vi "get_trigger.vi"(8 "error in (no error)":errorcluster, 11 "DAQmxWriteSignals in":refnum<class "SignalWriterMM140725DAQmx.lvclass">) -> (0 "error out":errorcluster, 1 "edge":T1, 2 "digital trigger line":tag, 3 "DAQmxWriteSignals out":refnum<class "SignalWriterMM140725DAQmx.lvclass">, 4 "trigger set?":bool)   [LabVIEW 2010, in "SignalWriterMM140725DAQmx.lvclass"]
uses:
  SignalWriterMM140725DAQmx.lvclass
  trigger_edge_enum.ctl
  SignalWriterMM140725DAQmx.lvclass/SignalWriterMM140725DAQmx.ctl
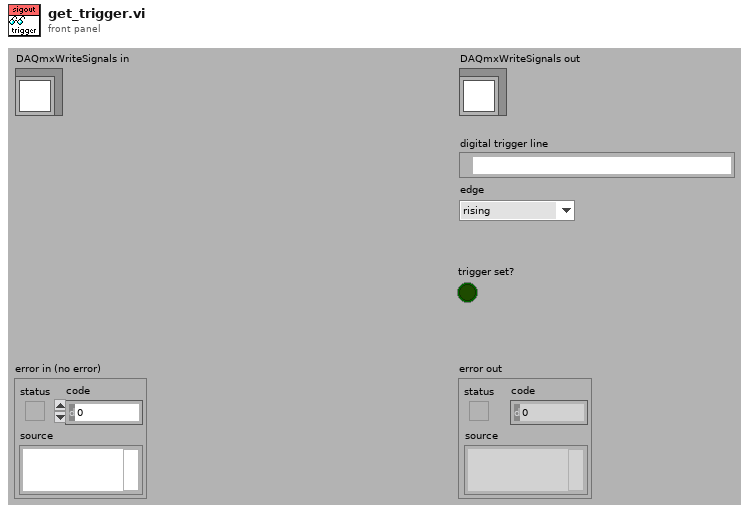
[diagram p1: front panel]
types:
  T1 = typedef "SignalWriterMM140725DAQmx.lvclass/trigger_edge_enum.ctl" = enum16{"rising", "falling"}
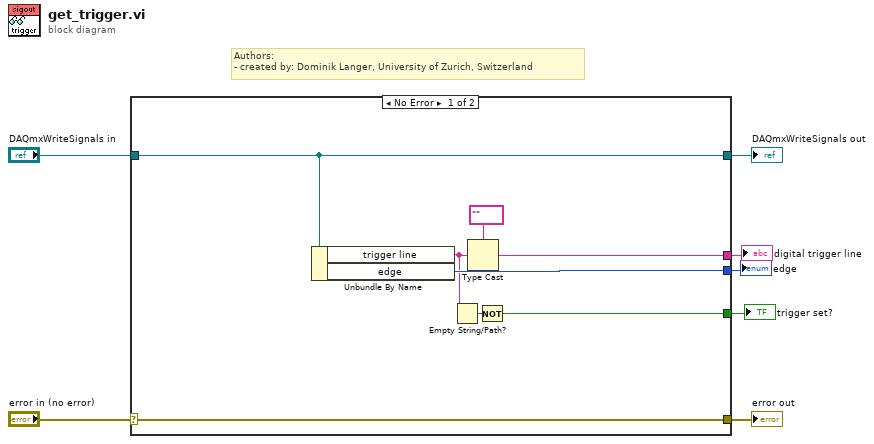
[diagram p0: block diagram]
diagram:
  # "Authors: \n- created by: Dominik Langer, University of Zurich, Switzerland"
  n1 = case shown="No Error" "error in (no error)" {
    selector: "error in (no error)" -> [w15 w17]
    tunnel: [w15 w17] -> w6
    tunnel: [w14 w16] -> w4
    tunnel: "DAQmxWriteSignals in" -> [w14 w16]
    tunnel: [w13 _] -> w3
    tunnel: [w12 _] -> w2
    tunnel: [w8 _] -> w1
    frame No Error {
      n2 = Unbundle By Name(w14) -> ("trigger line"=w10:string, "edge"=w13:T1)
      n3 = Empty String/Path?(string/path=w10) -> (empty?=w9:bool)
      n4 = Type Cast(type=tag "" ("digital trigger line"), x=w10) -> (*(type *) &x=w12:tag)
      n5 = Not(x=w9) -> (.not. x?=w8:bool)
    }
    frame Error {
    }
  }
  "error out" <- w6
  "DAQmxWriteSignals out" <- w4
  "digital trigger line" <- w2
  "edge" <- w3
  "trigger set?" <- w1
